vi "PathPlanner_PathConstraints_IsNull.vi"(11 "PathPlannerConstraints":T1) -> (3 "IsNull":bool)   [LabVIEW 2019, in "PathPlanner24.lvlib"]
doc: "Return indication that the PathConstraints data definition isn't null (not defined)\n\nInputs:\n - PathPlannerConstraints - cluster - Path Constraints definition to evaluate.\n\nOutputs:\n - IsNull - boolean - TRUE if definition is NULL."
uses:
  PathPlanner24.lvlib
  TypeDef/PathPlannerPathConstraints.ctl
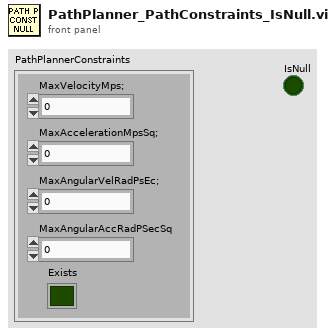
[diagram p1: front panel]
types:
  T1 = typedef "PathPlanner24.lvlib/PathPlannerPathConstraints.ctl" = cluster{"MaxVelocityMps;":dbl, "MaxAccelerationMpsSq;":dbl, "MaxAngularVelRadPsEc;":dbl, "MaxAngularAccRadPSecSq":dbl, "Exists":bool}
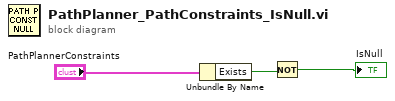
[diagram p0: block diagram]
diagram:
  n1 = Unbundle By Name("PathPlannerConstraints") -> ("Exists"=w2:bool)
  n2 = Not(x=w2) -> (.not. x?=→"IsNull":bool)
